vi "Create Transfer Configuration.vi"(7 "base transfer name (transfer)":string="transfer", 8 "non-random type (DBL)":T1=enum."DBL", 9 "random types? (F)":bool, 11 "channel count per transfer":i32) -> (3 "transfer configuration":T2)   [LabVIEW 2017]
uses:
  Built/DSF.Engine.lvlibp/Shared/Typedefs/DSF.Shared.Refactor.Typedefs.Transfer Configuration.ctl
  Built/DSF.Engine.lvlibp/Shared/Typedefs/DSF.Shared.Typedefs.Byte Order.ctl
  Built/DSF.Engine.lvlibp/Shared/Typedefs/DSF.Shared.Refactor.Typedefs.Channel Array Configuration.ctl
  Built/DSF.Engine.lvlibp/Shared/Typedefs/DSF.Shared.Typedefs.Data Type.ctl
  Built/DSF.Engine.lvlibp
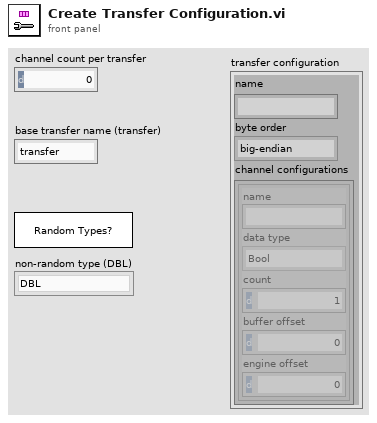
[diagram p1: front panel]
types:
  T1 = typedef "DSF.Engine.lvlibp/DSF.Shared.Typedefs.Data Type.ctl" = enum8{"Bool", "SGL", "DBL", "I8", "I16", "I32", "I64", "U8", "U16", "U32", "U64"}
  T2 = typedef "DSF.Engine.lvlibp/DSF.Shared.Refactor.Typedefs.Transfer Configuration.ctl" = cluster{"name":string, "byte order":T3, "channel configurations":T4[]}
  T3 = typedef "DSF.Engine.lvlibp/DSF.Shared.Typedefs.Byte Order.ctl" = enum8{"big-endian", "little-endian"}
  T4 = typedef "DSF.Engine.lvlibp/DSF.Shared.Refactor.Typedefs.Channel Array Configuration.ctl" = cluster{"name":string, "data type":T1, "count":u64, "buffer offset":u64, "engine offset":u64}
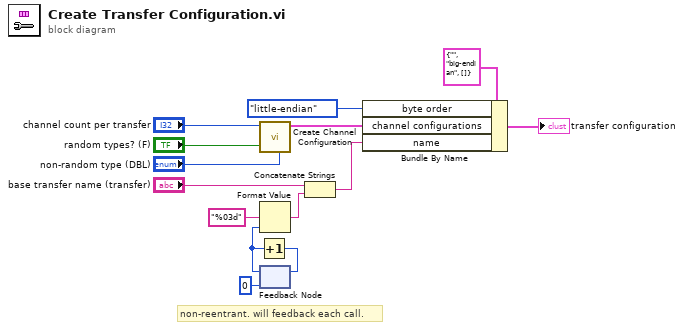
[diagram p0: block diagram]
diagram:
  # "non-reentrant. will feedback each call."
  n1 = call "Create Channel Configuration.vi"("non-random type (DBL)"="non-random type (DBL)", "random types? (F)"="random types? (F)", "channel count"="channel count per transfer") -> ("channel configurations"=w4:T4[])  [unwired: 7 in, 1 out]
  n2 = feedback #1(0) -> (w10:i32)
  n3 = Increment(x=w10) -> (x+1=w11:i32)
  n4 = Format Value(format string="%03d", value (0)=w10) -> (output string=w5:string)  [unwired: 1 in]
  n5 = feedback-in #1(w11) -> ()
  n6 = Concatenate Strings("base transfer name (transfer)", w5) -> (w3:string)
  n7 = Bundle By Name(cluster=T2 {"name"="", "byte order"=enum."big-endian", "channel configurations"=[]} ("Transfer Configuration"), "byte order"=DSF.Shared.Typedefs.Byte_Order."little-endian", "channel configurations"=w4, "name"=w3) -> (→"transfer configuration":T2)
